vi "FalconSwerveVelocityConversion.vi"(1 "Velocity (Raw Sensor Units per 100 ms)":i32) -> (0 "Velocity (ft/s)":dbl)   [LabVIEW 2019]
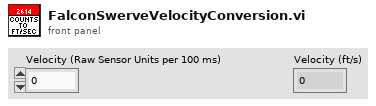
[diagram p1: front panel]
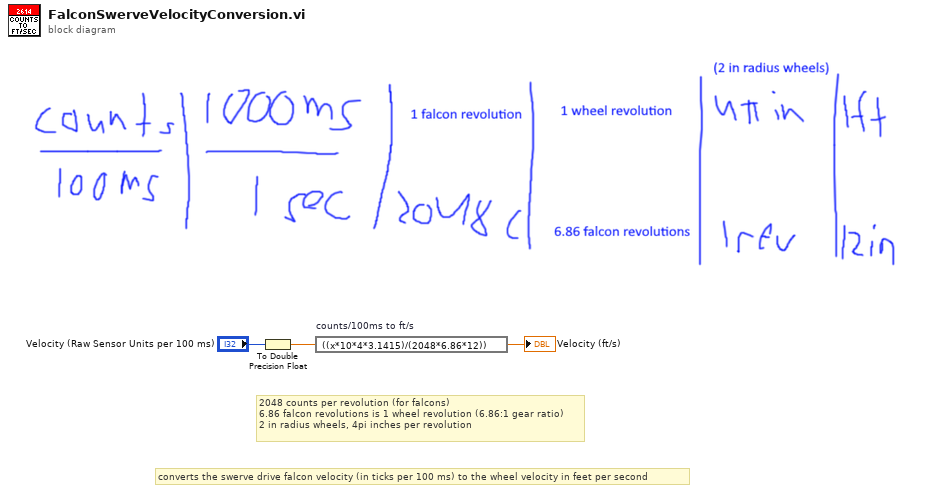
[diagram p0: block diagram]
diagram:
  # "converts the swerve drive falcon velocity (in ticks per 100 ms) to the wheel velocity in feet per second"
  # "2048 counts per revolution (for falcons)\n6.86 falcon revolutions is 1 wheel revolution (6.86:1 gear ratio)\n2 in radius wheels, 4pi inches per revolution"
  n1 = To Double Precision Float(number="Velocity (Raw Sensor Units per 100 ms)") -> (double precision float=w2:dbl)
  n2 = expression code="((x*10*4*3.1415)/(2048*6.86*12))" "counts/100ms to ft/s"(w2) -> (→"Velocity (ft/s)":dbl)
